vi "Get Code Generation Information.vi"(8 "error in (no error)":errorcluster, 11 "RIO Target in":refnum<class "RIO Target.lvclass">) -> (0 "error out":errorcluster, 2 "Bus Information Array":T1[](array[typedef]), 3 "RIO Target out":refnum<class "RIO Target.lvclass">)   [LabVIEW 2014, in "RIO Target.lvclass"]
uses:
  RIO Target.lvclass
  Scripting/Initialization Scripting/State Machine/Controls/Bus Information.ctl
  Scripting/Initialization Scripting/State Machine/Controls/Device Information.ctl
  Scripting/Initialization Scripting/State Machine/Controls/Pin Information.ctl
  <vilib>/NI/Configuration Framework/Node/NISE_CEF_Node.lvclass/NISE_CEF_Node.ctl
  Bus/Bus.lvclass
  Bus Configuration/Bus Configuration.lvclass
  Bus Configuration/Bus Configuration.lvclass/Bus Configuration.ctl
  <vilib>/NI/Configuration Framework/Node/NISE_CEF_Node.lvclass
  Scripting/Initialization Scripting/Initialization and IO Node Scripting.lvlib
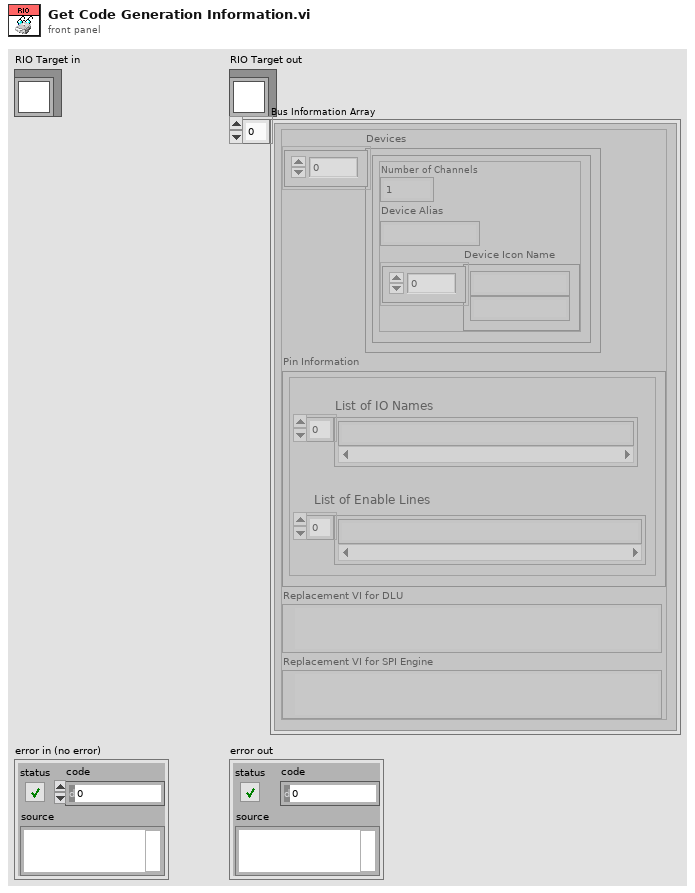
[diagram p1: front panel]
types:
  T1 = typedef "Initialization and IO Node Scripting.lvlib/Bus Information.ctl" = cluster{"Devices":T2[], "Pin Information":T3, "Replacement VI for DLU":path, "Replacement VI for SPI Engine":path}
  T2 = typedef "Device Information.ctl" = cluster{"Number of Channels":i32, "Device Alias":string, "Device Icon Name":string[]}
  T3 = typedef "Pin Information.ctl" = cluster{"List of IO Names":string[], "List of Enable Lines":string[]}
  T4 = typedef "NISE_CEF_Node.lvclass/NodeRef.ctl" = refnum<data-value>
  T5 = typedef "Bus Configuration.lvclass/SPI Configuration.ctl" = cluster{"SCLK":string, "MOSI":string, "MISO":string}
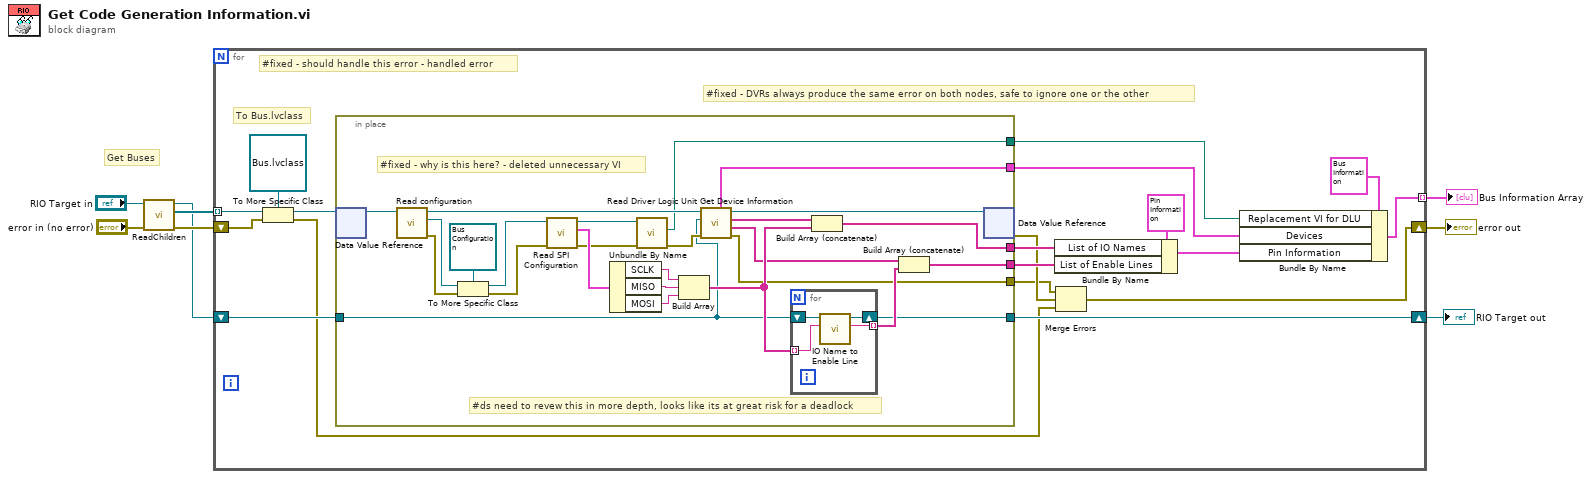
[diagram p0: block diagram]
diagram:
  # "Get Buses"
  n1 = call <vilib>:"ReadChildren.vi"("error in"="error in (no error)", "node in"="RIO Target in") -> ("error out"=w3:errorcluster, "output array"=w5:T4[], "node out"=w2:refnum<class "RIO Target.lvclass">)  [unwired: 7 in]
  n2 = for {
    tunnel: w5 -> [w26] mode=indexing
    shift-right: [w10] -> w8
    shift-left: w3 -> [w23]
    tunnel: [w22] -> w7 mode=indexing
    shift-right: [w13] -> w1
    shift-left: w2 -> [w18]
    # "#fixed - should handle this error - handled error"
    # "#fixed - DVRs always produce the same error on both nodes, safe to ignore one or the other"
    # "To Bus.lvclass"
    n3 = To More Specific Class(target class=refnum<data-value> refnum ("data value reference"), reference=w26, error in=w23) -> (specific class reference=w24:refnum<data-value>, error out=w11:errorcluster)
    n4 = in-place {
      in-place-border: w18 -> [w30]
      in-place-border: [w36] -> w17
      in-place-border: [w35] -> w16
      in-place-border: [w34] -> w15
      in-place-border: [w32] -> w14
      in-place-border: [w31] -> w13
      in-place-border: [w27] -> w9
      # "#fixed - why is this here? - deleted unnecessary VI"
      # "#ds need to revew this in more depth, looks like its at great risk for a deadlock"
      n5 = in-place-dvr #1(w24) -> (w52:refnum<class "Bus.lvclass">)  [unwired: 1 out]
      n6 = call-dynamic "Read configuration.vi"("Bus in"=w52) -> ("error out"=w47:errorcluster, "configuration"=w51:refnum<class "NISE_CEF_serializable configuration.lvclass">, "Bus out"=w46:refnum<class "Bus.lvclass">)  [unwired: 8 in]
      n7 = To More Specific Class(target class=refnum<class "Bus Configuration.lvclass"> refnum ("Bus Configuration.lvclass"), reference=w51, error in=w47) -> (specific class reference=w49:refnum<class "Bus Configuration.lvclass">, error out=w45:errorcluster)
      n8 = call "Read SPI Configuration.vi"("error in (no error)"=w45, "Bus Configuration in"=w49) -> ("error out"=w29:errorcluster, "SPI Configuration"=w48:T5, "Bus Configuration out"=w28:refnum<class "Bus Configuration.lvclass">)  [unwired: 7 in]
      n9 = Unbundle By Name(w48) -> ("SCLK"=w44:string, "MISO"=w43:string, "MOSI"=w42:string)
      n10 = call "Read Driver Logic Unit.vi"("error in (no error)"=w29, "Bus Configuration in"=w28) -> ("error out"=w33:errorcluster, "Driver Logic Unit"=w32:path)  [unwired: 7 in, 1 out]
      n11 = Build Array(w44, w43, w42) -> (w40:string[])
      n12 = call "Get Device Information.vi"("error in"=w33, "RIO Target in"=w30, "Bus in"=w46) -> ("error out"=w27:errorcluster, "Enable Lines"=w38:string[], "Chip Select Lines"=w41:string[], "Bus out"=w37:refnum<class "Bus.lvclass">, "Device Information Array"=w34:T2[])  [unwired: 4 in]
      n13 = for {
        shift-right: [w55] -> w31
        shift-left: w30 -> [w56]
        tunnel: [w54] -> w39 mode=indexing
        tunnel: w40 -> [w53] mode=indexing
        n14 = call-dynamic "IO Name to Enable Line.vi"("IO Name"=w53, "RIO Target in"=w56) -> ("Enable Line"=w54:string, "RIO Target out"=w55:refnum<class "RIO Target.lvclass">)  [unwired: 7 in, 1 out]
      }
      n15 = Build Array (concatenate)(w41, w40) -> (w36:string[])
      n16 = Build Array (concatenate)(w38, w39) -> (w35:string[])
      n17 = in-place-dvr #1(w37) -> (w12:errorcluster)  [unwired: 1 out]
    }
    n18 = Bundle By Name(cluster=T3 {"List of IO Names"=["sbRIO-9651 Socket\\PMOD1_Pin4_out", "sbRIO-9651 Socket\\PMOD1_Pin3_in", "sbRIO-9651 Socket\\PMOD1_Pin2_out", "sbRIO-9651 Socket\\PMOD1_Pin1_out"], "List of Enable Lines"=["sbRIO-9651 Socket\\PMOD1_Pin4_enable", "sbRIO-9651 Socket\\PMOD1_Pin3_enable", "sbRIO-9651 Socket\\PMOD1_Pin2_enable", "sbRIO-9651 Socket\\PMOD1_Pin1_enable"]} ("Pin Information"), "List of IO Names"=w17, "List of Enable Lines"=w16) -> (w19:T3)
    n19 = Merge Errors(w9, w12, w11) -> (w10:errorcluster)
    n20 = Bundle By Name(cluster=T1 {"Devices"=[], "Pin Information"={"List of IO Names"=["sbRIO-9651 Socket\\PMOD1_Pin4_out", "sbRIO-9651 Socket\\PMOD1_Pin3_in", "sbRIO-9651 Socket\\PMOD1_Pin2_out", "sbRIO-9651 Socket\\PMOD1_Pin1_out"], "List of Enable Lines"=["sbRIO-9651 Socket\\PMOD1_Pin4_enable", "sbRIO-9651 Socket\\PMOD1_Pin3_enable", "sbRIO-9651 Socket\\PMOD1_Pin2_enable", "sbRIO-9651 Socket\\PMOD1_Pin1_enable"]}, "Replacement VI for DLU"=path "E:/Documents/Projects/SPIAPI/Scripting Code  with State Machine 01_16_15 - Integrating with GUI/Test/Replacement.vi", "Replacement VI for SPI Engine"=path ""} ("Bus Information"), "Replacement VI for DLU"=w14, "Devices"=w15, "Pin Information"=w19) -> (w22:T1)
  }
  "error out" <- w8
  "RIO Target out" <- w1
  "Bus Information Array" <- w7
